vi "_PC_Pub_Display_StringMangement.vi"(4 "Clear error (T)":bool=TRUE, 5 "Reset(F)":bool, 6 "Max rows (last num)":i32, 7 "Is a new row (T)":bool=TRUE, 8 "error in (no error)":errorcluster, 9 "New string":string, 11 "String reference in":refnum<vi>) -> (0 "error out":errorcluster, 3 "reference out":refnum<vi>)   [LabVIEW 2016]
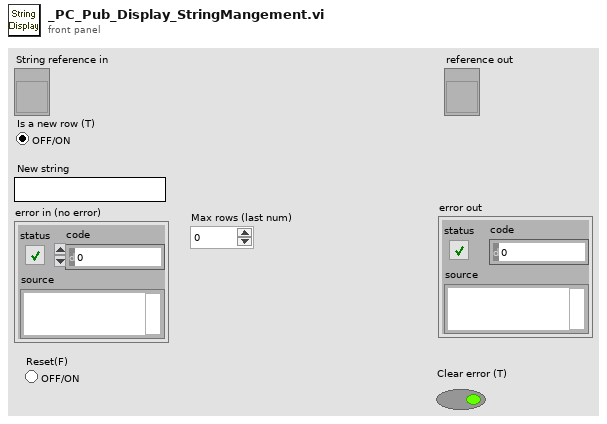
[diagram p1: front panel]
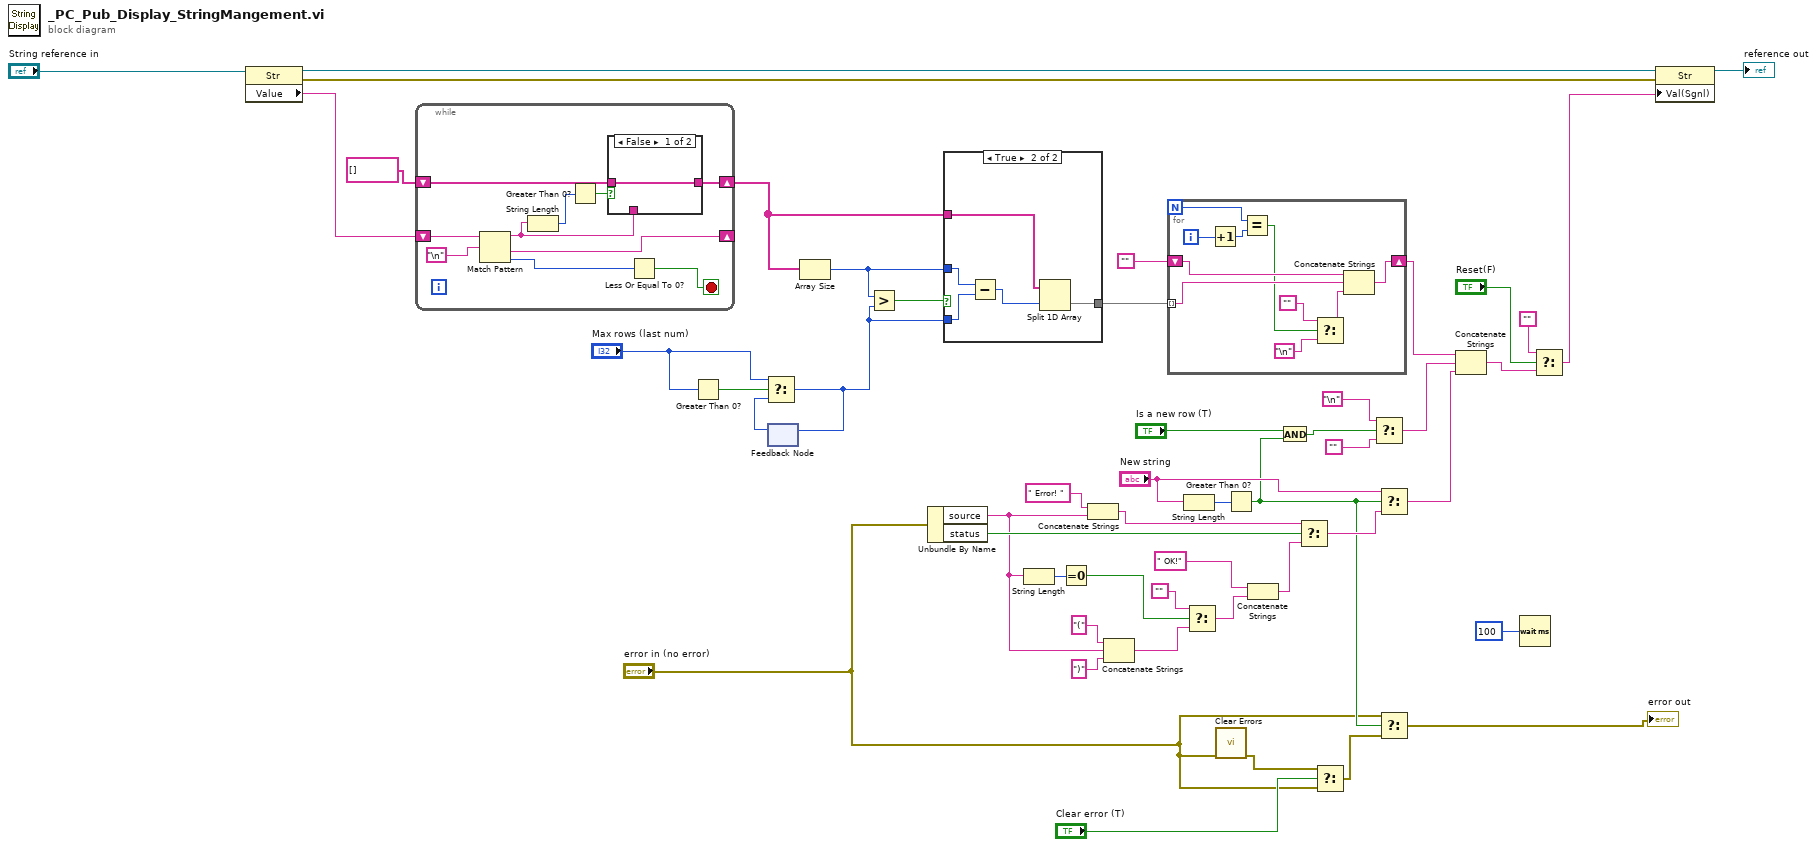
[diagram p0: block diagram]
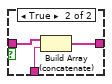
[diagram p3: hidden frame]
diagram:
  n1 = property class="Str"(reference="String reference in") -> (reference out=w45:refnum<vi>, error out=w44:errorcluster, "Value"=w41:string)  [unwired: 1 in]
  n2 = while {
    shift-right: [w57] -> _
    shift-left: w41 -> [w58]
    shift-right: [w56] -> w36
    shift-left: string[] [] -> [w55]
    stop <- w54 stop-if-true
    n3 = Match Pattern(string=w58, regular expression="\n") -> (before substring=w52:string, after substring=w57:string, offset past match=w53:i32)  [unwired: 1 in, 1 out]
    n4 = String Length(string=w52) -> (length=w51:i32)
    n5 = Greater Than 0?(x=w51) -> (x > 0?=w50:bool)
    n6 = case shown="False" w50 {
      tunnel: [w60 w63] -> w56
      tunnel: w55 -> [w60 w62]
      tunnel: w52 -> [_ w61]
      frame False {
      }
      frame True {
        n7 = Build Array (concatenate)(w62, w61) -> (w63:string[])
      }
    }
    n8 = Less Or Equal To 0?(x=w53) -> (x <= 0?=w54:bool)
  }
  n9 = Greater Than 0?(x="Max rows (last num)") -> (x > 0?=w40:bool)
  n10 = feedback #1() -> (w38:i32)  [unwired: 1 in]
  n11 = Select(t="Max rows (last num)", s=w40, f=w38) -> (s? t:f=w37:i32)
  n12 = feedback-in #1(w37) -> ()
  n13 = Array Size(array=w36) -> (size(s)=w47:i32)
  n14 = Greater?(x=w47, y=w37) -> (0:w48:bool)
  n15 = Unbundle By Name("error in (no error)") -> ("source"=w19:string, "status"=w27:bool)
  n16 = case shown="True" w48 {
    tunnel: w36 -> [w64 w66]
    tunnel: w47 -> [_ w69]
    tunnel: w37 -> [_ w68]
    tunnel: [w64 w65] -> w35
    frame False {
    }
    frame True {
      n17 = Subtract(x=w69, y=w68) -> (x-y=w67:i32)
      n18 = Split 1D Array(array=w66, index=w67) -> (second subarray=w65:string[])  [unwired: 1 out]
    }
  }
  n19 = String Length(string=w19) -> (length=w18:i32)
  n20 = Equal To 0?(x=w18) -> (x = 0?=w17:bool)
  n21 = Concatenate Strings(" Error! " ("string"), w19) -> (w25:string)
  n22 = Concatenate Strings("(" ("string"), w19, ")" ("string")) -> (w16:string)
  n23 = for {
    N -> [w74]
    tunnel: w35 -> [w79] mode=indexing
    shift-right: [w78] -> w31
    shift-left: "" -> [w77]
    i -> [w76]
    n24 = Increment(x=w76) -> (x+1=w75:i32)
    n25 = Equal?(x=w74, y=w75) -> (x = y?=w70:bool)
    n26 = Select(t="", s=w70, f="\n") -> (s? t:f=w72:string)
    n27 = Concatenate Strings(w77, w79, w72) -> (w78:string)
  }
  n28 = String Length(string="New string") -> (length=w30:i32)
  n29 = Select(t="", s=w17, f=w16) -> (s? t:f=w14:string)
  n30 = call <vilib>:"Clear Errors.vi"("error in (no error)"="error in (no error)") -> ("error out"=w4:errorcluster)  [unwired: 5 in, 1 out]
  n31 = Greater Than 0?(x=w30) -> (x > 0?=w7:bool)
  n32 = Concatenate Strings(" OK!" ("f"), w14) -> (w12:string)
  n33 = And(x="Is a new row (T)", y=w7) -> (x .and. y?=w23:bool)
  n34 = Select(t=w25, s=w27, f=w12) -> (s? t:f=w26:string)
  n35 = Select(t=w4, s="Clear error (T)", f="error in (no error)") -> (s? t:f=w2:errorcluster)
  n36 = Select(t="\n", s=w23, f="") -> (s? t:f=w32:string)
  n37 = Select(t="New string", s=w7, f=w26) -> (s? t:f=w28:string)
  n38 = Select(t="error in (no error)", s=w7, f=w2) -> (s? t:f=→"error out":errorcluster)
  n39 = Concatenate Strings(w31, w32, w28) -> (w11:string)
  n40 = Wait (ms)(milliseconds to wait=u32 100) -> ()  [unwired: 1 out]
  n41 = Select(t="", s="Reset(F)", f=w11) -> (s? t:f=w10:string)
  n42 = property class="Str"(reference=w45, error in=w44, "Val(Sgnl)"=w10) -> (reference out=→"reference out":refnum<vi>)  [unwired: 1 out]
